vi "Read Topic Info.vi"(11 "Topic in":refnum<class "Topic.lvclass">) -> (0 "Last Publication Time":timestamp, 1 "Last Topic Value":variant, 2 "Name":string, 3 "Type":string)   [LabVIEW 2015, in "Mediator.lvlib" / "Topic.lvclass"]
doc: "<License>\nCopyright © 2017 Composed Systems, LLC | All rights reserved\nwww.composed.io\n\nAuthor: Ethan Stern <ethan.stern@composed.io>\n\nThis software is provided \"AS IS\" WITHOUT WARRANTIES, either express or implied, AND IS FOR EDUCATIONAL PURPOSES ONLY.\n</License>"
uses:
  Topic.lvclass
  Topic.lvclass/Topic.ctl
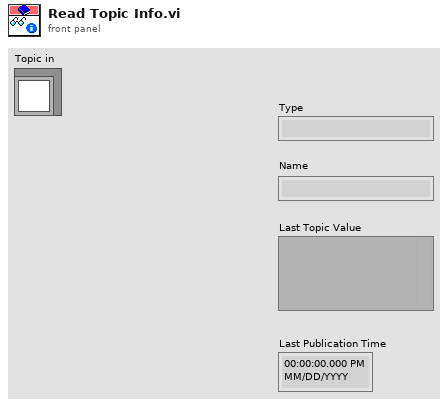
[diagram p1: front panel]
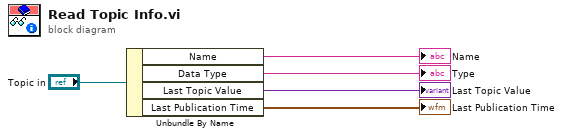
[diagram p0: block diagram]
diagram:
  n1 = Unbundle By Name("Topic in") -> ("Name"=→"Name":string, "Data Type"=→"Type":string, "Last Topic Value"=→"Last Topic Value":variant, "Last Publication Time"=→"Last Publication Time":timestamp)
